vi "Write ALR_index.vi"(8 "error in (no error)":errorcluster, 10 "ALR_index":i32[](array[numeric]), 11 "valve_VCH in":refnum<class "valve_VCH.lvclass">) -> (0 "error out":errorcluster, 3 "valve_VCH out":refnum<class "valve_VCH.lvclass">)   [LabVIEW 2019, in "valve_VCH.lvclass"]
uses:
  valve_VCH.lvclass
  valve_VCH.lvclass/valve_VCH.ctl
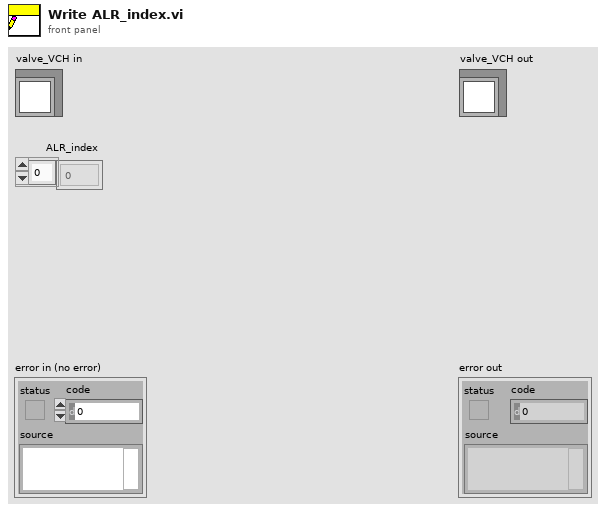
[diagram p1: front panel]
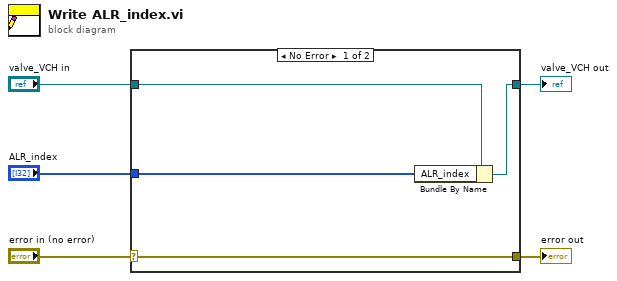
[diagram p0: block diagram]
diagram:
  n1 = case shown="No Error" "error in (no error)" {
    selector: "error in (no error)" -> [w9 w10]
    tunnel: [w9 w10] -> w4
    tunnel: [w7 w11] -> w2
    tunnel: "valve_VCH in" -> [w8 w11]
    tunnel: "ALR_index" -> [w6 _]
    frame No Error {
      n2 = Bundle By Name(cluster=w8, "ALR_index"=w6) -> (w7:refnum<class "valve_VCH.lvclass">)
    }
    frame Error {
    }
  }
  "error out" <- w4
  "valve_VCH out" <- w2
